vi "ESTOP.vi"(0 "ESTOP References":T1) -> ()   [LabVIEW 2011]
uses:
  C:/Program Files (x86)/National Instruments/LabVIEW 2011/user.lib/aerotech/8.2/Bin/Aerotech.A3200.dll
  Program Files (x86)/National Instruments/LabVIEW 2011/user.lib/aerotech/8.2/Bin/Aerotech.A3200.dll
  <vilib>/DAQmx/write.llb/DAQmx Write (Digital Bool 1Line 1Point).vi
  <vilib>/DAQmx/write.llb/DAQmx Write (Digital 1D Bool 1Chan 1Samp).vi
  <vilib>/DAQmx/miscellaneous.llb/DAQmx Fill In Error Info.vi
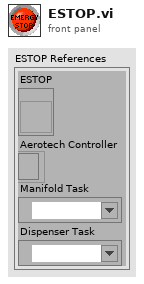
[diagram p1: front panel]
types:
  T1 = cluster{"ESTOP":refnum<vi>, "Aerotech Controller":refnum<k24>, "Manifold Task":refnum<k21>, "Dispenser Task":refnum<k21>}
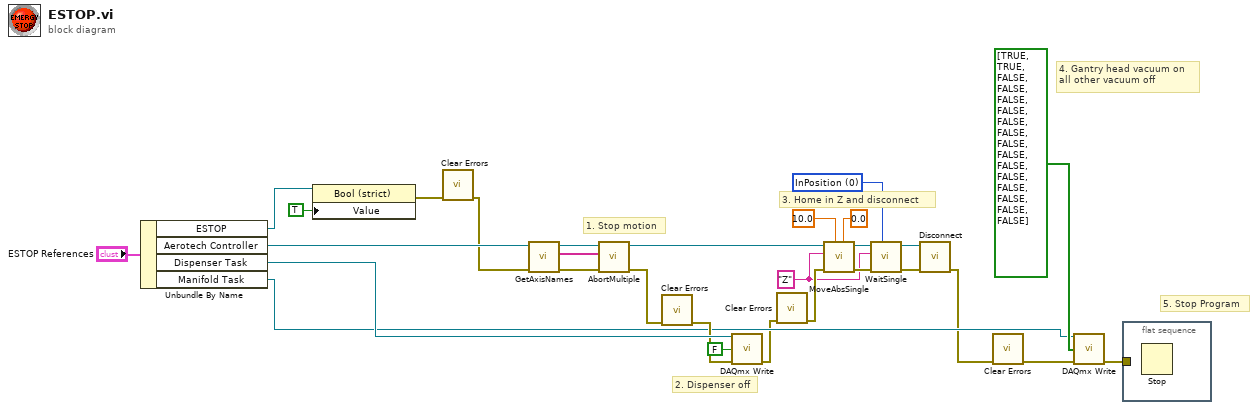
[diagram p0: block diagram]
diagram:
  w8 = 0 items=["InPosition", "MoveDone"] ("wait option?")
  w10 = "Z" ("axis name")
  # "3. Home in Z and disconnect"
  # "5. Stop Program"
  # "1. Stop motion"
  # "2. Dispenser off"
  # "4. Gantry head vacuum on\nall other vacuum off"
  n1 = Unbundle By Name("ESTOP References") -> ("ESTOP"=w28:refnum<vi>, "Aerotech Controller"=w5:refnum<k24>, "Dispenser Task"=w26:refnum<k21>, "Manifold Task"=w19:refnum<k21>)
  n2 = property class="Bool (strict)"(reference=w28, "Value"=TRUE) -> (error out=w20:errorcluster)  [unwired: 1 in, 1 out]
  n3 = call <vilib>:"Clear Errors.vi"("error in (no error)"=w20) -> ("error out"=w1:errorcluster)  [unwired: 6 in]
  n4 = call <userlib>:"GetAxisNames.vi"("error in (no error)"=w1, "controller in"=w5) -> ("error out"=w2:errorcluster, "axis names"=w3:string[], "controller out"=w4:refnum<k24>)  [unwired: 7 in]
  n5 = call <userlib>:"AbortMultiple.vi"("error in (no error)"=w2, "axis names"=w3, "controller in"=w4) -> ("error out"=w6:errorcluster, "controller out"=w7:refnum<k24>)  [unwired: 7 in]
  n6 = call <vilib>:"Clear Errors.vi"("error in (no error)"=w6) -> ("error out"=w25:errorcluster)  [unwired: 6 in]
  n7 = call-poly <vilib>:"DAQmx Write.vi"("task/channels in"=w26, "data"=FALSE, "error in"=w25) -> ("error out"=w18:errorcluster)  [unwired: 10 in, 2 out]
  n8 = call <vilib>:"Clear Errors.vi"("error in (no error)"=w18) -> ("error out"=w14:errorcluster)  [unwired: 6 in]
  n9 = call <userlib>:"MoveAbsSingle.vi"("position"=0.0, "speed"=10.0, "error in (no error)"=w14, "axis name"=w10, "controller in"=w7) -> ("error out"=w11:errorcluster, "controller out"=w13:refnum<k24>)  [unwired: 5 in]
  n10 = call <userlib>:"WaitSingle.vi"("wait option?"=w8, "error in (no error)"=w11, "axis name"=w10, "controller in"=w13) -> ("error out"=w9:errorcluster, "controller out"=w12:refnum<k24>)  [unwired: 5 in, 1 out]
  n11 = call <userlib>:"Disconnect.vi"("error in (no error)"=w9, "controller"=w12) -> ("error out"=w17:errorcluster)  [unwired: 9 in]
  n12 = call <vilib>:"Clear Errors.vi"("error in (no error)"=w17) -> ("error out"=w24:errorcluster)  [unwired: 6 in]
  n13 = call-poly <vilib>:"DAQmx Write.vi"("task/channels in"=w19, "data"=bool[] [TRUE, TRUE, FALSE, FALSE, FALSE, FALSE, FALSE, FALSE, FALSE, FALSE, FALSE, FALSE, FALSE, FALSE, FALSE, FALSE], "error in"=w24) -> ("error out"=w21:errorcluster)  [unwired: 10 in, 2 out]
  n14 = flat-sequence {
    tunnel: w21 -> [_]
    frame #0 {
      n15 = Stop() -> ()  [unwired: 1 in]
    }
  }
